vi "FGV_ListConfig.vi"(7 "Set":bool, 8 "error in (no error)":errorcluster caption="错误输入（无错误）", 11 "Config":T1={"TimeFormat"=0, "ID Format"=0, "Data Format"=0, "ListLen"=1000} {"ListLen" min=1000 max=100000; "Data Format" items=["十六进制", "十进制", "二进制", "ASCII码"]; "ID Format" items=["十六进制", "十进制"]; "TimeFormat" items=["系统时间", "时间戳(s)"]}) -> (0 "error out":errorcluster caption="错误输出", 3 "Config out":T1={"TimeFormat"=0, "ID Format"=0, "Data Format"=0, "ListLen"=1000} {"ListLen" min=1000 max=100000; "Data Format" items=["十六进制", "十进制", "二进制", "ASCII码"]; "ID Format" items=["十六进制", "十进制"]; "TimeFormat" items=["系统时间", "时间戳(s)"]})   [LabVIEW 2018, in "CAN FD.lvlib"]
uses:
  CAN FD.lvlib
  Typedef/Config.ctl
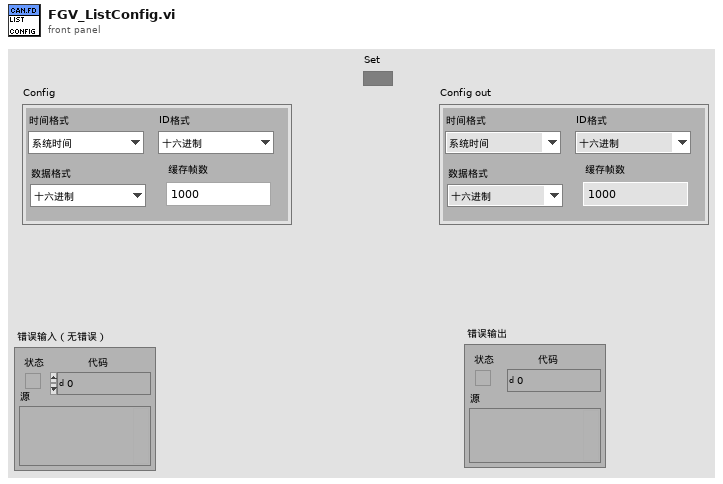
[diagram p1: front panel]
types:
  T1 = typedef "CAN FD.lvlib/Config.ctl" = cluster{"TimeFormat":u16, "ID Format":u16, "Data Format":u16, "ListLen":u32}
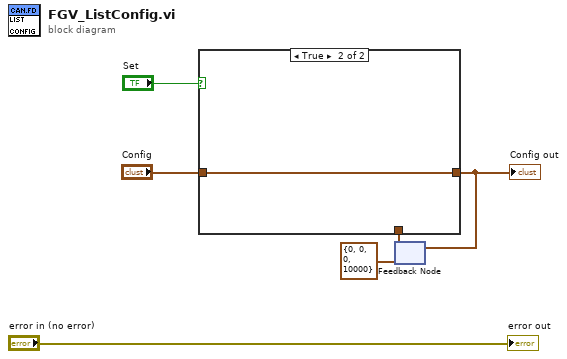
[diagram p0: block diagram]
diagram:
  n1 = feedback #1(T1 {"TimeFormat"=0, "ID Format"=0, "Data Format"=0, "ListLen"=10000} ("Config out")) -> (w2:T1)
  n2 = case shown="True" "Set" {
    tunnel: "Config" -> [_ w8]
    tunnel: [w7 w8] -> w3
    tunnel: w2 -> [w7 _]
    frame False {
    }
    frame True {
    }
  }
  "Config out" <- w3
  n3 = feedback-in #1(w3) -> ()
  "error out" <- "error in (no error)"
